vi "Get LakeShore 370 Resistance_GPIB.vi"(8 "error in (no error)":errorcluster, 9 "Seconds between samples":dbl=1.0 format="%_4f", 10 "Channels to scan (empty - don't use scanner option)":i32[](array[numeric]), 11 "GPIB Adress":i16) -> (0 "error out":errorcluster, 2 "Resistance":dbl[](array[numeric]))   [LabVIEW 2015]
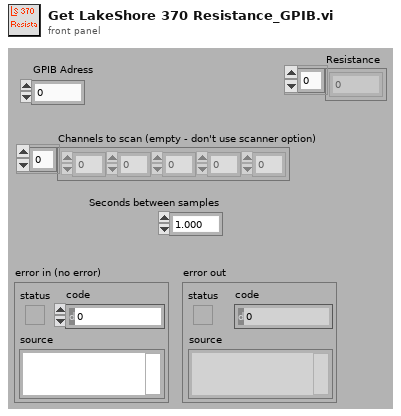
[diagram p1: front panel]
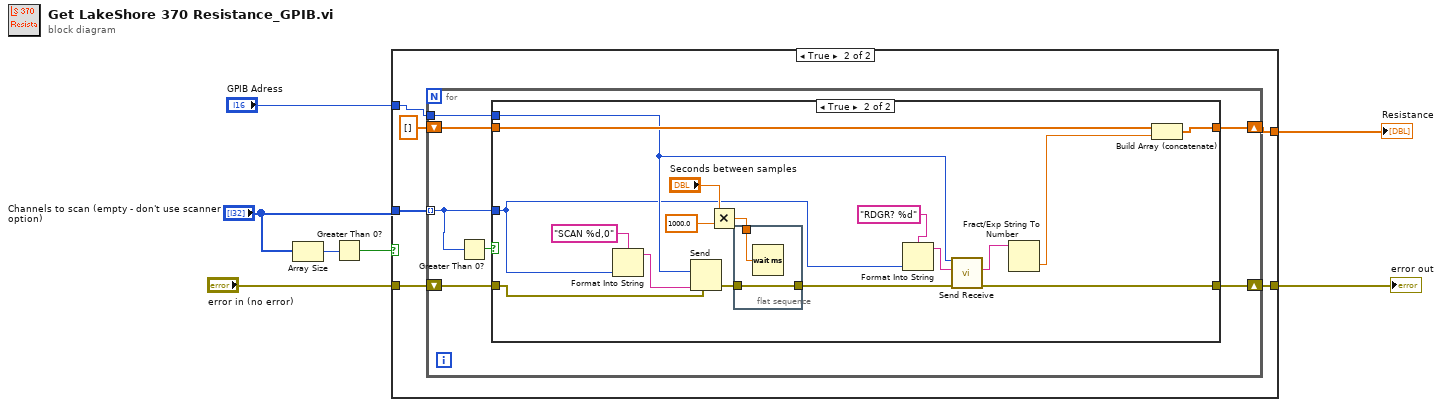
[diagram p0: block diagram]
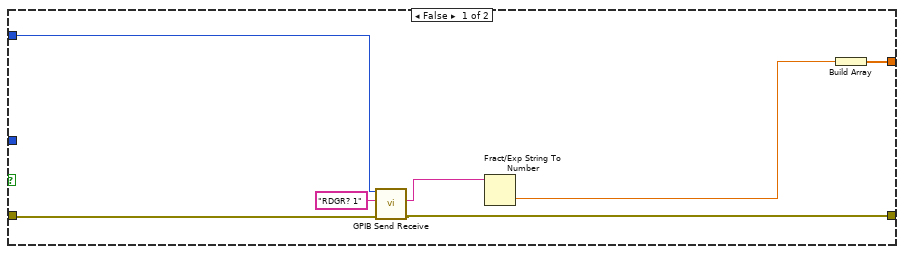
[diagram p2: hidden frame]
diagram:
  n1 = Array Size(array="Channels to scan (empty - don't use scanner option)") -> (size(s)=w7:i32)
  n2 = Greater Than 0?(x=w7) -> (x > 0?=w6:bool)
  n3 = case shown="True" w6 {
    tunnel: "Channels to scan (empty - don't use scanner option)" -> [_ w20]
    tunnel: [w14 w19] -> w2
    tunnel: "error in (no error)" -> [w11 w18]
    tunnel: [w10 w17] -> w1
    tunnel: "GPIB Adress" -> [w9 w15]
    frame False {
      n4 = call "GPIB Send Receive.vi"("error in (no error)"=w11, "data string in"="RDGR? 1", "GPIB Adress"=w9) -> ("error out"=w10:errorcluster, "data string out"=w13:string)  [unwired: 6 in, 1 out]
      n5 = Fract/Exp String To Number(string=w13) -> (number=w8:dbl)  [unwired: 4 out]
      n6 = Build Array(w8) -> (w14:dbl[])
    }
    frame True {
      n7 = for {
        tunnel: w20 -> [w21] mode=indexing
        shift-right: [w24] -> w19
        shift-left: dbl[] [] -> [w23]
        shift-right: [w25] -> w17
        shift-left: w18 -> [w27]
        tunnel: w15 -> [w22]
        n8 = Greater Than 0?(x=w21) -> (x > 0?=w26:bool)
        n9 = case shown="True" w26 {
          tunnel: w21 -> [_ w31]
          tunnel: w27 -> [w28 w39]
          tunnel: [w28 w35] -> w25
          tunnel: [w29 w43] -> w24
          tunnel: w23 -> [w29 w42]
          tunnel: w22 -> [_ w34]
          frame False {
          }
          frame True {
            n10 = Format Into String(format string="SCAN %d,0", w31) -> (resulting string=w40:string)  [unwired: 2 in, 1 out]
            n11 = Send(2:w34, 4:w39, 5:w40) -> (8:w38:errorcluster)  [unwired: 4 out]
            n12 = Multiply(x="Seconds between samples", y=1000.0) -> (x*y=w44:dbl)
            n13 = flat-sequence {
              tunnel: [w47] -> w36
              tunnel: w44 -> [w48]
              tunnel: w38 -> [w47]
              frame #0 {
                n14 = Wait (ms)(milliseconds to wait=w48) -> ()  [unwired: 1 out]
              }
            }
            n15 = Format Into String(format string="RDGR? %d" ("data string in"), w31) -> (resulting string=w33:string)  [unwired: 2 in, 1 out]
            n16 = call-poly "Send Receive.vi"("error in (no error)"=w36, "data string in"=w33, "GPIB Adress"=w34) -> ("error out"=w35:errorcluster, "data string out"=w37:string)  [unwired: 6 in, 1 out]
            n17 = Fract/Exp String To Number(string=w37) -> (number=w30:dbl)  [unwired: 4 out]
            n18 = Build Array (concatenate)(w42, w30) -> (w43:dbl[])
          }
        }
      }
    }
  }
  "error out" <- w1
  "Resistance" <- w2
